vi "Set Items (Anything).vi"(8 "error in (no error)":errorcluster, 9 "Value":variant[](array[variant]), 10 "Item Paths":string[](array[string]), 11 "CycloneDX SBOM in":refnum<class "CycloneDX JSON.lvclass">) -> (0 "error out":errorcluster, 3 "CycloneDX SBOM out":refnum<class "CycloneDX JSON.lvclass">)   [LabVIEW 2017, in "LabVIEW CycloneDX SBOM.lvlib" / "CycloneDX JSON.lvclass"]
doc: "Adds multiple items (any LV datatype) at the specified JSON path."
uses:
  CycloneDX JSON.lvclass
  CycloneDX JSON.lvclass/CycloneDX JSON.ctl
  c57fa5db-63f9-4e40-b316-3a77e1eb2573.vi
  <vilib>/JDP Science/JSONtext/Variant to JSON Text.vi
  <vilib>/JDP Science/JSONtext/Get all Object Items.vi
  <vilib>/JDP Science/JSONtext/Set Multiple Object Items.vi
  <vilib>/JDP Science/JSONtext/JSONtext.lvlib
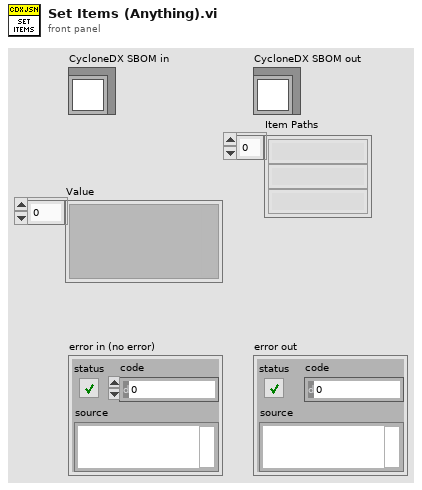
[diagram p1: front panel]
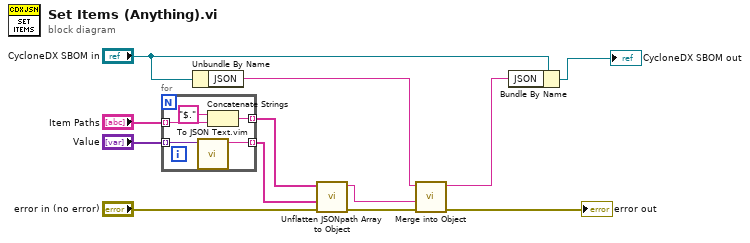
[diagram p0: block diagram]
diagram:
  n1 = for {
    tunnel: "Value" -> [w17] mode=indexing
    tunnel: [w16] -> w8 mode=indexing
    tunnel: "Item Paths" -> [w15] mode=indexing
    tunnel: [w13] -> w1 mode=indexing
    n2 = call "To JSON Text.vim"("Anything"=w17) -> ("<JSON>"=w16:string)  [unwired: 9 in, 1 out]
    n3 = Concatenate Strings("$." ("string"), w15) -> (w13:string)
  }
  n4 = Unbundle By Name("CycloneDX SBOM in") -> ("JSON"=w6:string)
  n5 = call <vilib>:"Unflatten JSONpath Array to Object.vi"("error in (no error)"="error in (no error)", "JSON Items"=w8, "$Paths"=w1) -> ("error out"=w10:errorcluster, "<JSON>"=w7:string)  [unwired: 7 in]
  n6 = call <vilib>:"Merge into Object.vi"("error in (no error)"=w10, "JSON Object to Merge"=w7, "JSON"=w6) -> ("error out"=→"error out":errorcluster, "<JSON>"=w4:string)  [unwired: 6 in]
  n7 = Bundle By Name(cluster="CycloneDX SBOM in", "JSON"=w4) -> (→"CycloneDX SBOM out":refnum<class "CycloneDX JSON.lvclass">)
